vi "MGI Average (DBL[][]).vi"(0 "Double[][]":dbl[][](array[numeric]), 1 "Ignore NaN? (F)":bool) -> (2 "Average":dbl)   [LabVIEW 2020]
doc: "This VI computes and returns the average value of the given array of doubles.\n\nAuthored by Shawn D. Walpole\nsupport@mooregoodideas.com\nwww.mooregoodideas.com\n\nCopyright (c) 2010, Moore Good Ideas, Inc.\n\nAll rights reserved.\n\nRedistribution and use in source and binary forms, with or without modification, are permitted provided that the following conditions are met:\n\n * Redistributions of source code must retain the above copyright notice, this list of conditions and the following disclaimer.\n * Redistributions in binary form must reproduce the above copyright notice, this list of conditions and the following disclaimer in the documentation and/or other materials provided with the distribution.\n * Neither the name of Moore Good Ideas, Inc. nor the names of its contributors may be used to endorse or promote products derived from this software without specific prior written permission.\n\nTHIS SOFTWARE IS PROVIDED BY THE COPYRIGHT HOLDERS AND CONTRIBUTORS \"AS IS\" AND ANY EXPRESS OR IMPLIED WARRANTIES, INCLUDING, BUT NOT LIMITED TO, THE IMPLIED WARRANTIES OF MERCHANTABILITY AND FITNESS FOR A PARTICULAR PURPOSE ARE DISCLAIMED. IN NO EVENT SHALL THE COPYRIGHT OWNER OR CONTRIBUTORS BE LIABLE FOR ANY DIRECT, INDIRECT, INCIDENTAL, SPECIAL, EXEMPLARY, OR CONSEQUENTIAL DAMAGES (INCLUDING, BUT NOT LIMITED TO, PROCUREMENT OF SUBSTITUTE GOODS OR SERVICES; LOSS OF USE, DATA, OR PROFITS; OR BUSINESS INTERRUPTION) HOWEVER CAUSED AND ON ANY THEORY OF LIABILITY, WHETHER IN CONTRACT, STRICT LIABILITY, OR TORT (INCLUDING NEGLIGENCE OR OTHERWISE) ARISING IN ANY WAY OUT OF THE USE OF THIS SOFTWARE, EVEN IF ADVISED OF THE POSSIBILITY OF SUCH DAMAGE."
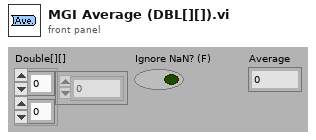
[diagram p1: front panel]
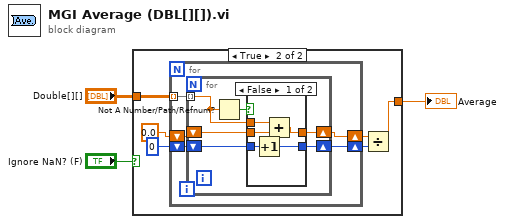
[diagram p0: block diagram]
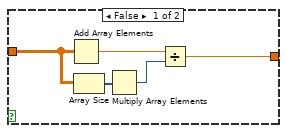
[diagram p2: hidden frame]
diagram:
  n1 = case shown="True" "Ignore NaN? (F)" {
    tunnel: "Double[][]" -> [w6 w12]
    tunnel: [w5 w9] -> w2
    frame False {
      n2 = Add Array Elements(numeric array=w6) -> (sum=w8:dbl)
      n3 = Array Size(array=w6) -> (size(s)=w7:i32[])
      n4 = Multiply Array Elements(1:w7) -> (0:w4:i32)
      n5 = Divide(x=w8, y=w4) -> (x/y=w5:dbl)
    }
    frame True {
      n6 = for {
        tunnel: w12 -> [w17] mode=indexing
        shift-right: [w15] -> w10
        shift-left: 0 -> [w19]
        shift-right: [w16] -> w11
        shift-left: 0.0 -> [w18]
        n7 = for {
          shift-right: [w20] -> w16
          shift-left: w18 -> [w22]
          shift-right: [w23] -> w15
          shift-left: w19 -> [w24]
          tunnel: w17 -> [w21] mode=indexing
          n8 = Not A Number/Path/Refnum?(number/path/refnum=w21) -> (NaN/Path/Refnum?=w25:bool)
          n9 = case shown="False" w25 {
            tunnel: w24 -> [w30 w31]
            tunnel: [w29 w31] -> w23
            tunnel: w22 -> [w28 w32]
            tunnel: w21 -> [w27 _]
            tunnel: [w26 w32] -> w20
            frame False {
              n10 = Increment(x=w30) -> (x+1=w29:i32)
              n11 = Add(x=w27, y=w28) -> (x+y=w26:dbl)
            }
            frame True {
            }
          }
        }
      }
      n12 = Divide(x=w11, y=w10) -> (x/y=w9:dbl)
    }
  }
  "Average" <- w2
